vi "Global Motors.vi"() -> ()   [LabVIEW 2014]
panel:
  in  "Initial Z":dbl
  out "M3 move Complete":bool
  in  "Motor 3":refnum<k7>
  out "Lines Progress":i64
  in  "Initial Y":dbl
  in  "Initial X":dbl
  in  "Y Line Time (mm/s)":dbl
  in  "X Line Time (mm/s)":dbl
  out "M2 move Complete":bool
  out "M1 move Complete":bool
  in  "Motor 2":refnum<k7>
  in  "Motor 1":refnum<k7>
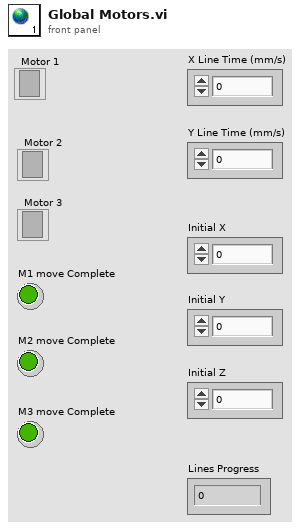
[diagram p1: front panel]
diagram:
